vi "init.vi"(8 "Error In":errorcluster, 10 "I2C Adres":u8=29 format="%.0x", 11 "LINX Ref":T1) -> (0 "Error Out":errorcluster, 3 "LINX Resource":T1)   [LabVIEW 2014]
doc: "Open the I2C master and initialize the MMA8452 accelerometer.\n\nIf the LINX device has more than one I2C master the logical first I2C master is channel 0, the next is channel 1, etc."
uses:
  <vilib>/MakerHub/LINX/Private/Type Defs/LINX Ref.ctl
  <vilib>/MakerHub/LINX/Private/Type Defs/Platform.ctl
  <vilib>/MakerHub/LINX/Private/Type Defs/Interface.ctl
  <vilib>/MakerHub/LINX/Private/Device/Type Defs/LINX Device Config.ctl
  <vilib>/MakerHub/LINX/Private/Device/Type Defs/TCP Config.ctl
  <vilib>/MakerHub/LINX/Private/Device/Type Defs/Channels.ctl
  <vilib>/MakerHub/LINX/Private/Local IO/LinxI2cWrite.vi
  <vilib>/MakerHub/LINX/Public/Utilities/Check Channel.vi
  <vilib>/MakerHub/LINX/Private/Local IO/Handle Errors.vi
  <vilib>/MakerHub/LINX/Private/Utilties/Generate Error.vi
  <vilib>/MakerHub/LINX/LMH-LINX.lvlib
  <vilib>/MakerHub/LINX/Private/Device/Device.lvlib
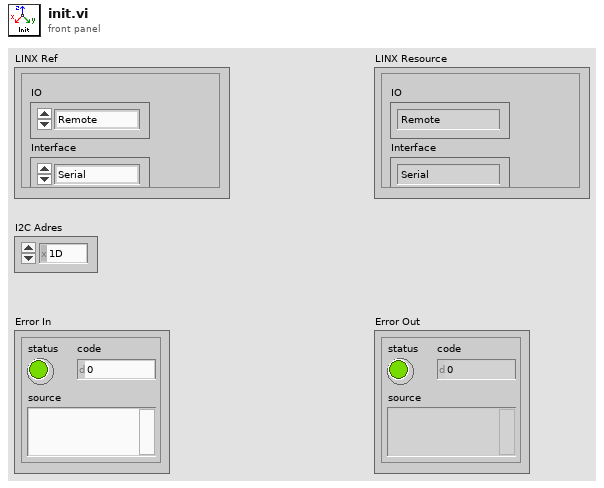
[diagram p1: front panel]
types:
  T1 = typedef "LMH-LINX.lvlib/LINX Ref.ctl" = cluster{"IO":T2, "Interface":T3, "LINX Device Config":T4}
  T2 = typedef "LMH-LINX.lvlib/Platform.ctl" = enum16{"Remote", "Local"}
  T3 = typedef "LMH-LINX.lvlib/Interface.ctl" = enum16{"Serial", "TCP"}
  T4 = typedef "LMH-LINX.lvlib/Device.lvlib/LINX Device Config.ctl" = cluster{"Interface":T3, "COM Port":refnum<visa-resource-name>, "TCP Configuration":T5, "Device Family":u8, "Device ID":u8, "Device Name":string, "TCP Ref":refnum<k5>, "Channels":T6}
  T5 = typedef "LMH-LINX.lvlib/Device.lvlib/TCP Config.ctl" = cluster{"IP Address":string, "Port":u16}
  T6 = typedef "LMH-LINX.lvlib/Channels.ctl" = cluster{"DI":u8[], "DO":u8[], "AI":u8[], "AO":u8[], "PWM":u8[], "QE":u8[], "UART":u8[], "I2C 2":u8[], "SPI":u8[], "CAN":u8[], "Servo":u8[], "AI Ref (V)":dbl, "AI Resolution (Bits)":u8, "AO Ref (V)":dbl, "AO Resolution (Bits)":u8}
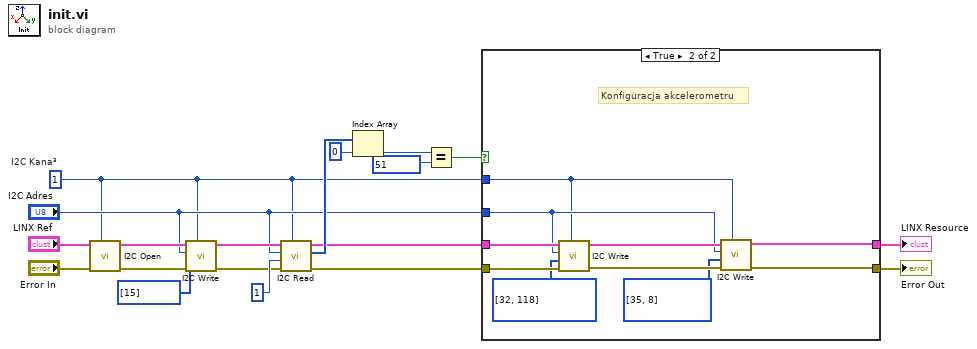
[diagram p0: block diagram]
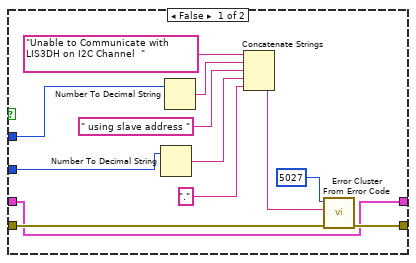
[diagram p2: hidden frame]
diagram:
  w2 = u8 1  # I2C Kana³
  n1 = call <vilib>:"I2C Open.vi"("I2C Channel (0)"=w2, "Error In"="Error In", "LINX Resource"="LINX Ref") -> ("Error Out"=w5:errorcluster, "LINX Resource"=w7:T1)  [unwired: 7 in]
  n2 = call <vilib>:"I2C Write.vi"("I2C Channel"=w2, "Error In"=w5, "Data"=u8[] [15], "I2C Slave Address (0)"="I2C Adres", "LINX Resource"=w7) -> ("Error Out"=w4:errorcluster, "LINX Resource"=w6:T1)  [unwired: 5 in]
  n3 = call <vilib>:"I2C Read.vi"("I2C Channel"=w2, "Error In"=w4, "Bytes To Read"=u8 1, "I2C Slave Address (0)"="I2C Adres", "LINX Resource"=w6) -> ("Error Out"=w11:errorcluster, "Data"=w16:u8[], "LINX Resource"=w10:T1)  [unwired: 4 in]
  n4 = Index Array(array=w16, index=0) -> (element=w18:u8)
  n5 = Equal?(x=w18, y=u8 51) -> (x = y?=w12:bool)
  n6 = case shown="True" w12 {
    tunnel: w11 -> [w25 w40]
    tunnel: w10 -> [w20 w41]
    tunnel: [w23 w35] -> w9
    tunnel: w2 -> [w22 w33]
    tunnel: "I2C Adres" -> [w21 w34]
    tunnel: [w20 w36] -> w8
    frame False {
      n7 = Number To Decimal String(number=w21) -> (decimal integer string=w30:string)  [unwired: 1 in]
      n8 = Number To Decimal String(number=w22) -> (decimal integer string=w28:string)  [unwired: 1 in]
      n9 = Concatenate Strings("Unable to Communicate with LIS3DH on I2C Channel  " ("error message (\"\")"), w28, " using slave address " ("string"), w30, "." ("string")) -> (w24:string)
      n10 = call <vilib>:"Error Cluster From Error Code.vi"("error in (no error)"=w25, "error message (\"\")"=w24, "error code (0)"=5027) -> ("error out"=w23:errorcluster)  [unwired: 6 in]
    }
    frame True {
      # "Konfiguracja akcelerometru"
      n11 = call <vilib>:"I2C Write.vi"("I2C Channel"=w33, "Error In"=w40, "Data"=u8[] [32, 118], "I2C Slave Address (0)"=w34, "LINX Resource"=w41) -> ("Error Out"=w37:errorcluster, "LINX Resource"=w38:T1)  [unwired: 5 in]
      n12 = call <vilib>:"I2C Write.vi"("I2C Channel"=w33, "Error In"=w37, "Data"=u8[] [35, 8], "I2C Slave Address (0)"=w34, "LINX Resource"=w38) -> ("Error Out"=w35:errorcluster, "LINX Resource"=w36:T1)  [unwired: 5 in]
    }
  }
  "LINX Resource" <- w8
  "Error Out" <- w9
